vi "FITS hdr gen row dbl.vi"(5 "Format":string, 9 "Comment":string, 10 "Value":dbl, 11 "Field":string) -> (3 "FITS Row":string)   [LabVIEW 2022 SP3]
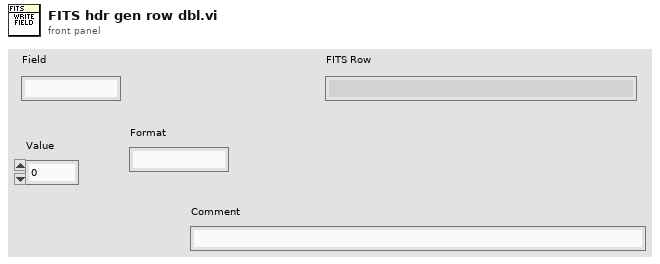
[diagram p1: front panel]
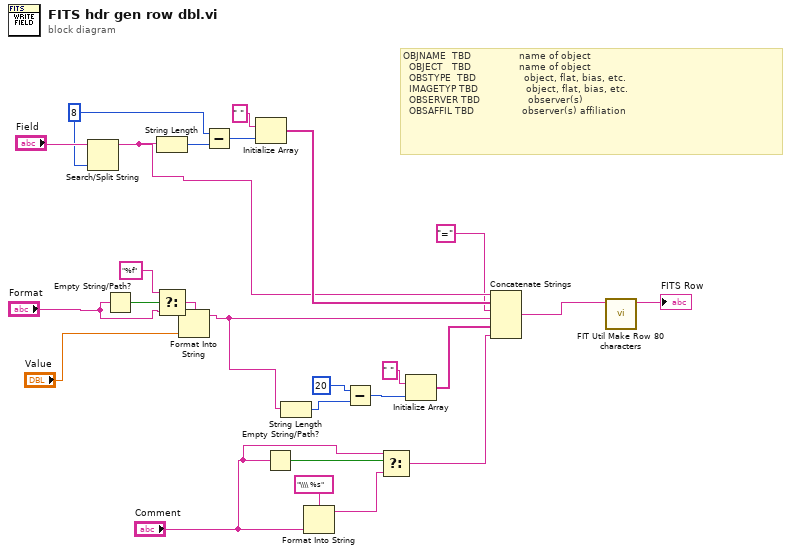
[diagram p0: block diagram]
diagram:
  w25 = 8
  # "OBJNAME  TBD                name of object\n  OBJECT   TBD                name of object\n  OBSTYPE  TBD                object, flat, bias, etc.\n  IMAGETYP TBD                object, flat, bias, etc.\n  OBSERVER TBD                observer(s) \n  OBSAFFIL TBD                observer(s) affiliation"
  n1 = Search/Split String(string="Field", offset (0)=w25) -> (substring before match=w2:string)  [unwired: 1 in, 2 out]
  n2 = Empty String/Path?(string/path="Format") -> (empty?=w16:bool)
  n3 = String Length(string=w2) -> (length=w24:i32)
  n4 = Select(t="%f", s=w16, f="Format") -> (s? t:f=w14:string)
  n5 = Format Into String(format string=w14, "Value") -> (resulting string=w9:string)  [unwired: 2 in, 1 out]
  n6 = Subtract(x=w25, y=w24) -> (x-y=w23:i32)
  n7 = Initialize Array(" ", w23) -> (w18:string[])
  n8 = Empty String/Path?(string/path="Comment") -> (empty?=w6:bool)
  n9 = String Length(string=w9) -> (length=w11:i32)
  n10 = Format Into String(format string="\\\\ %s", "Comment") -> (resulting string=w4:string)  [unwired: 2 in, 1 out]
  n11 = Subtract(x=20, y=w11) -> (x-y=w10:i32)
  n12 = Select(t="Comment", s=w6, f=w4) -> (s? t:f=w3:string)
  n13 = Initialize Array(" ", w10) -> (w8:string[])
  n14 = Concatenate Strings(w2, w18, "=" ("string"), w9, w8, w3) -> (w17:string)
  n15 = call "FIT Util Make Row 80 characters.vi"("Row"=w17) -> ("Row with 80 char"=→"FITS Row":string)  [unwired: 10 in]
